vi "Execute Git Command.vi"(6 "Arguments":string[](array[string]), 7 "Command":string="merge" caption="Command (merge)", 8 "error in (no error)":errorcluster, 9 "File Paths":path[](array[path]), 10 "Git Implementation":refnum<class "Git Implementation.lvclass">, 11 "Git-Merger in":refnum<class "Merge-Delegate.lvclass">) -> (0 "error out":errorcluster, 2 "CMD Return":T1, 3 "Git-Merger out":refnum<class "Merge-Delegate.lvclass">)   [LabVIEW 2017, in "Git-LabVIEW.lvlib" / "Merge-Delegate.lvclass"]
doc: "This VI provides a wrapper for the Git Implementation \"Execute Command\" method, which is Community scope.\nIt is used to allow the Git-Merge class hierarchy to act as delegates for the purpose of merging branches."
uses:
  Merge-Delegate.lvclass
  Implementation/Git Implementation.lvclass
  CMD Return.ctl
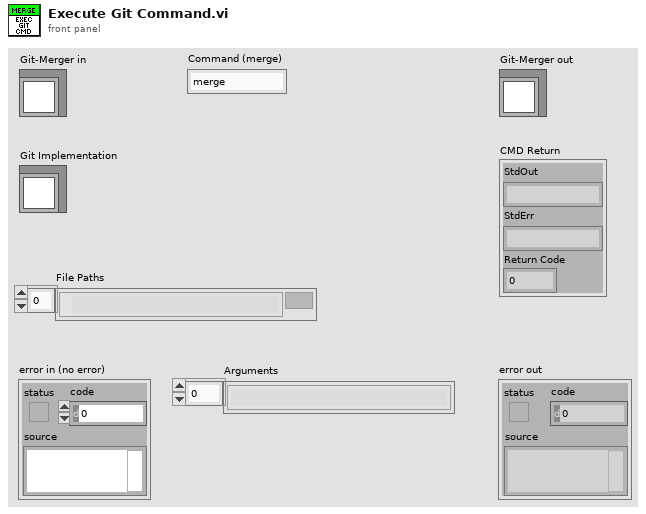
[diagram p1: front panel]
types:
  T1 = typedef "Git-LabVIEW.lvlib/Merge-Delegate.lvclass/CMD Return.ctl" = cluster{"StdOut":string, "StdErr":string, "Return Code":i32}
  T2 = typedef "Git-LabVIEW.lvlib/Git Implementation.lvclass/CMD Return.ctl" = cluster{"StdOut":string, "StdErr":string, "Return Code":i32}
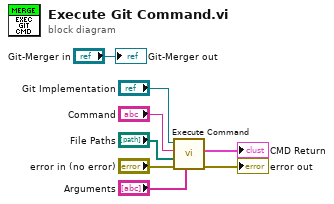
[diagram p0: block diagram]
diagram:
  n1 = call "Execute Command.vi"("Arguments"="Arguments", "error in (no error)"="error in (no error)", "File Paths"="File Paths", "Command"="Command", "Git Implementation in"="Git Implementation") -> ("error out"=→"error out":errorcluster, "CMD Return"=→"CMD Return":T2)  [unwired: 4 in, 1 out]
  "Git-Merger out" <- "Git-Merger in"
